vi "laser_controller.vi"() -> ()   [LabVIEW 2014]
uses:
  <vilib>/Instr/_visa.llb/VISA Configure Serial Port (Instr).vi
  <vilib>/FieldPoint/Polymorphic Read.llb/FP Read (Float Array).vi
  <vilib>/FieldPoint/Polymorphic Write.llb/FP Write (Float).vi
panel:
  in  "Ignore Ethernal":bool
  in  "Change Power?":bool
  out "TEC Setpoint":dbl=39.06 format="%#_13g"
  out "Power":dbl(graph)=89.68
  in  "DISABLE":bool
  in  "ENABLE":bool
  in  "LEVEL CONTROL, 0-100 (%)":dbl(knob) scale=0.0..100.0
  out "Temp":dbl(graph)=38.91
  in  "Which Temp?":enum16{"ETH", "PUMP", "PCB", "AMP", "CASE"}(ring)
  out "Temp Stable":bool=TRUE
  out "Software Enabled":bool=TRUE
  out "Hardware Enabled":bool=TRUE
  in  "Ethernal COM Port":refnum<visa-resource-name>="COM3"
  in  "LEVEL CONTROL, 0-10 (W)":dbl(knob) scale=0.0..10.0
  in  "AMPLIFIER ENABLE":bool=TRUE
  out "Pre-amp Mon (Amps)":dbl=5.782406330108643 format="%#_3g"
  out "Temp Mon (deg C)":dbl(slide)=24.883191287517548 scale=0.0..50.0
  out "Mid Power Mon (Volts, no-cal)":dbl=4.550704002380371 format="%#_3g"
  out "Out Power Mon (Volts, no-cal)":dbl=1.5106858015060425 format="%#_3g"
  out "+5 Vdc Out":dbl=4.966402530670166 format="%#_3g"
  out "Power-Amp Pump Current (Amps)":dbl format="%#_3g"
  out "Seed Mon (Volts, no-cal)":dbl=4.966084957122803 format="%#_3g"
  out "Back Refl. Mon (Volts, no-cal)":dbl=0.007061874959617853 format="%#_3g"
  out "Power Supply Fault":bool=TRUE
  out "Temp. Fault":bool=TRUE
  out "Back Refl. Fault":bool=TRUE
  out "Seed Power Fault":bool=TRUE
  out "Master Fault":bool=TRUE
  in  "Controller Stop":bool
  in  "Control Rate (ms)":u32=1000
  # "ORBITS SEED LASER"
  # "NUFERN FIBER AMPLIFIER"
  # "STATUS"
  # "FAULT STATUS"
  # "MONITORS"
  # "OFF STATUS"
  # "ON STATUS"
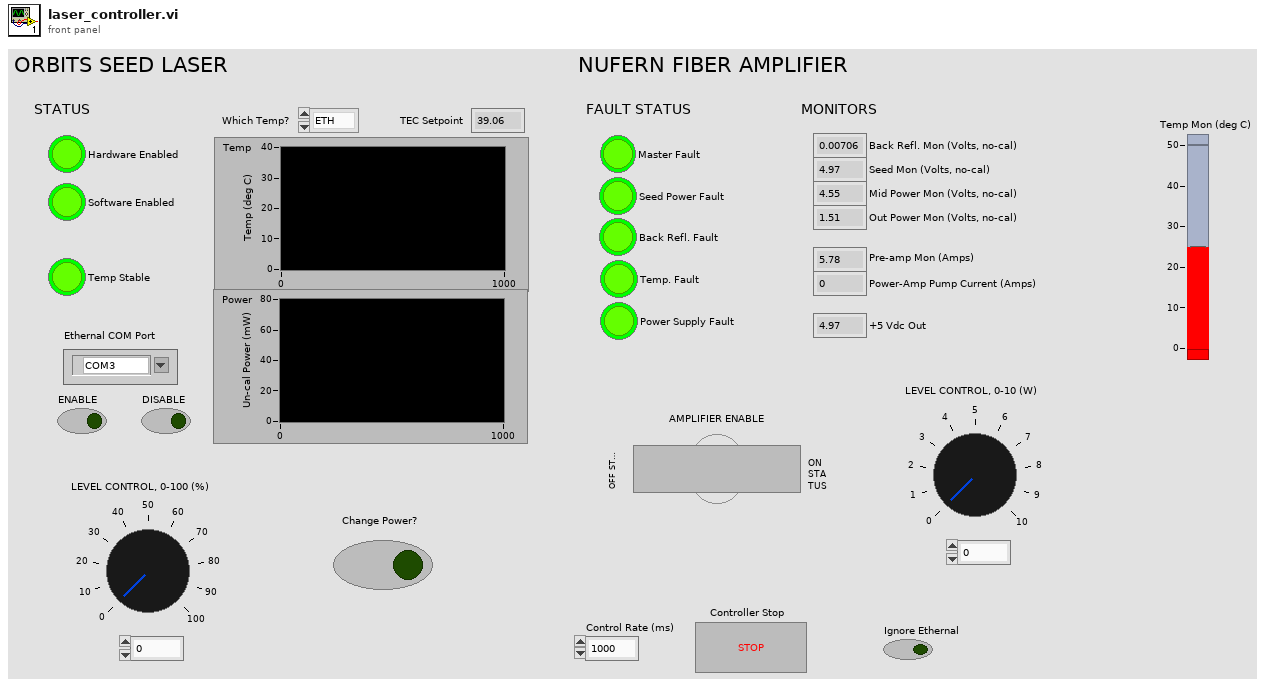
[diagram p1: front panel]
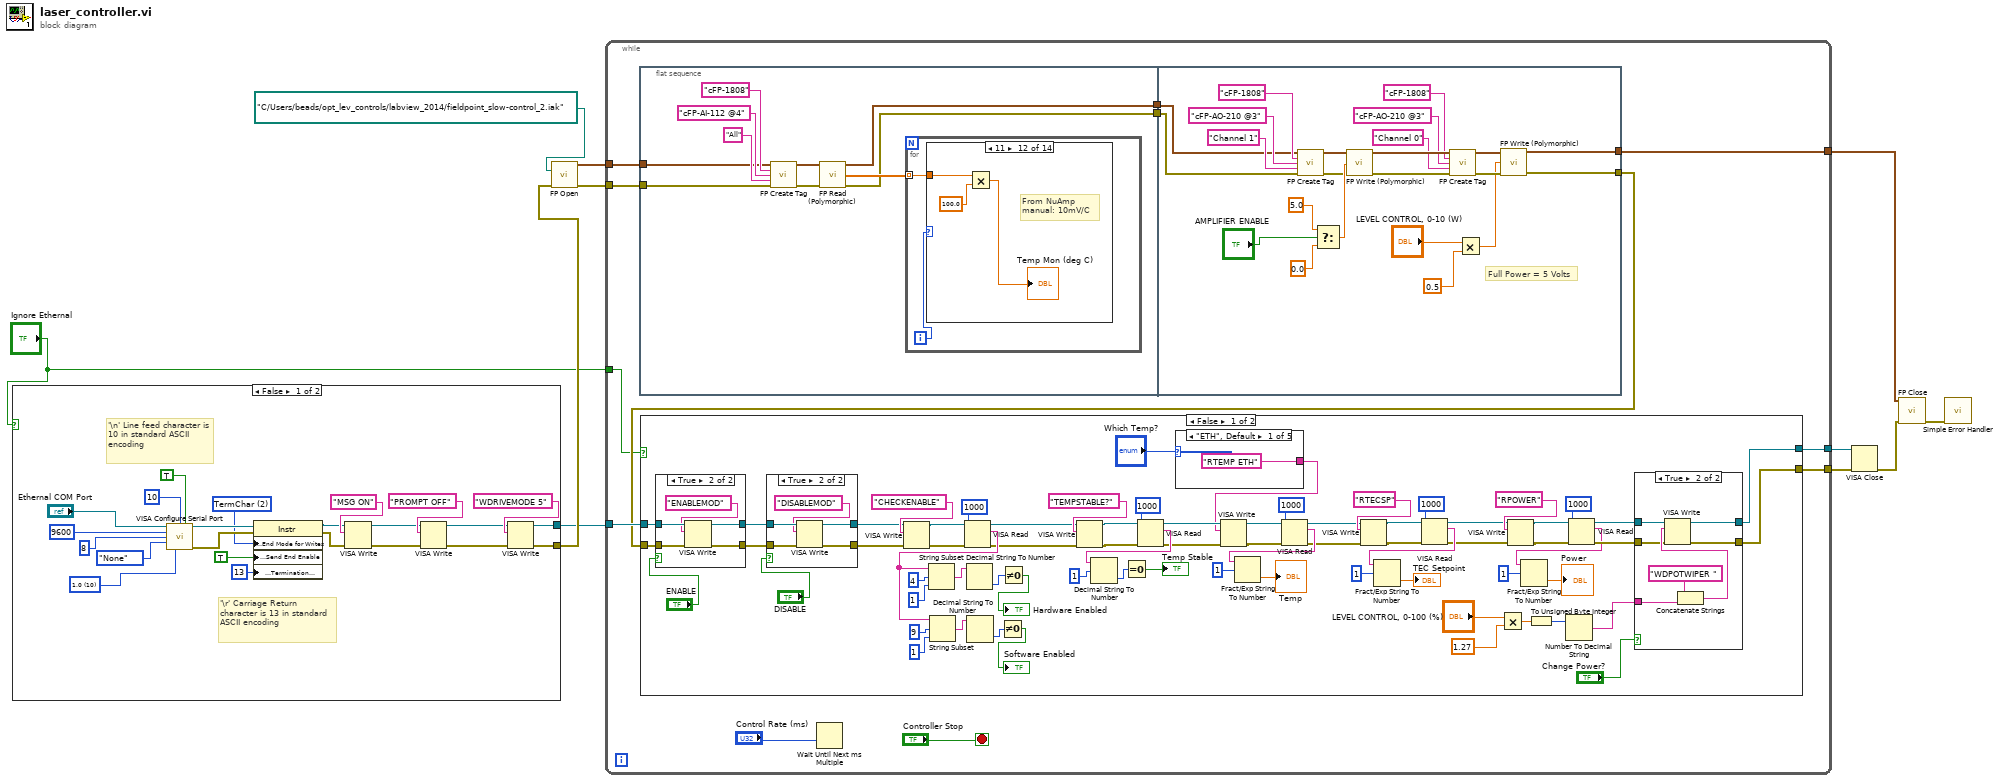
[diagram p0: block diagram]
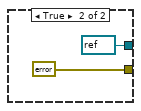
[diagram p2: hidden frame]
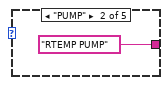
[diagram p6: hidden frame]
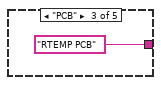
[diagram p7: hidden frame]
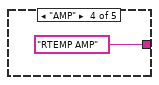
[diagram p8: hidden frame]
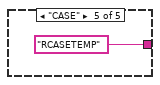
[diagram p9: hidden frame]
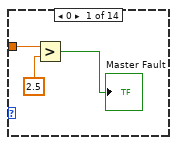
[diagram p11: hidden frame]
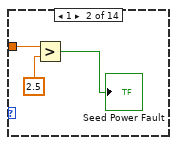
[diagram p12: hidden frame]
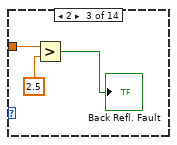
[diagram p13: hidden frame]
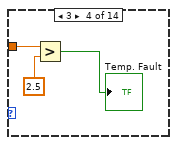
[diagram p14: hidden frame]
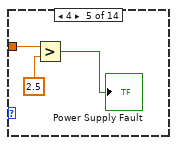
[diagram p15: hidden frame]
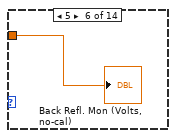
[diagram p16: hidden frame]
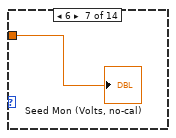
[diagram p17: hidden frame]
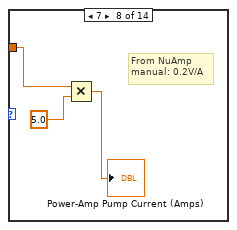
[diagram p18: hidden frame]
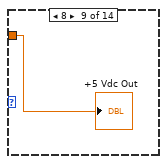
[diagram p19: hidden frame]
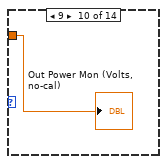
[diagram p20: hidden frame]
diagram:
  n1 = case shown="False" "Ignore Ethernal" {
    tunnel: [w13 errorcluster {"status"=FALSE, "code"=0, "source"=""} ("error out")] -> w3
    tunnel: [w12 refnum<visa-resource-name> refnum ("VISA resource name out")] -> w2
    frame False {
      w17 = u16 10 items=["1.0"=10, "1.5"=15, "2.0"=20] ("stop bits (10: 1 bit)")
      w31 = u16 2 items=["None", "LastBit", "TermChar", "Break"] ("Serial Settings:Serial End Mode for Writes")
      # "'\\r' Carriage Return character is 13 in standard ASCII encoding"
      # "'\\n' Line feed character is 10 in standard ASCII encoding"
      n2 = call-poly "VISA Configure Serial Port"("VISA resource name"="Ethernal COM Port", "termination char\n(0xA = '\\n' = LF)"=u8 10, "Enable Termination\nChar (T)"=TRUE, "baud rate (9600)"=u32 9600, "data bits (8)"=u16 8, "parity (0:none)"=enum16{"None", "Odd", "Even", "Mark", "Space"}."None", "stop bits (10: 1 bit)"=w17) -> ("VISA resource name out"=w33:refnum<visa-resource-name>, "error out"=w34:errorcluster)  [unwired: 3 in, 4 out]
      n3 = property class="Instr"(reference=w33, error in=w34, "Serial Settings:End Mode for Writes"=w31, "Message Based Settings:Send End Enable"=TRUE, "Message Based Settings:Termination Character"=13) -> (reference out=w22:refnum<visa-resource-name>, error out=w23:errorcluster)
      n4 = VISA Write(VISA resource name=w22, write buffer="MSG ON" ("Enable 2"), error in (no error)=w23) -> (VISA resource name out=w20:refnum<visa-resource-name>, error out=w19:errorcluster)  [unwired: 1 out]
      n5 = VISA Write(VISA resource name=w20, write buffer="PROMPT OFF" ("Enable 2"), error in (no error)=w19) -> (VISA resource name out=w15:refnum<visa-resource-name>, error out=w14:errorcluster)  [unwired: 1 out]
      n6 = VISA Write(VISA resource name=w15, write buffer="WDRIVEMODE 5" ("Enable 2"), error in (no error)=w14) -> (VISA resource name out=w12:refnum<visa-resource-name>, error out=w13:errorcluster)  [unwired: 1 out]
    }
    frame True {
    }
  }
  n7 = call <vilib>:"FP Open.vi"("iak file path"=path "C:/Users/beads/opt_lev_controls/labview_2014/fieldpoint_slow-control_2.iak", "error in (no error)"=w3) -> ("FP refnum out"=w11:cluster{"server refnum":u32, "tag refnum":u32}, "error out"=w10:errorcluster)  [unwired: 12 in]
  n8 = while {
    tunnel: w11 -> [w46]
    tunnel: w10 -> [w45]
    tunnel: [w42] -> w8
    tunnel: w2 -> [w39]
    tunnel: [w41] -> w5
    tunnel: [w40] -> w4
    tunnel: "Ignore Ethernal" -> [w37]
    stop <- "Controller Stop" stop-if-true
    n9 = flat-sequence {
      tunnel: w46 -> [w153]
      tunnel: w45 -> [w152]
      tunnel: [w151] -> w44
      tunnel: [w150] -> w43
      tunnel: w44 -> [w210]
      tunnel: w43 -> [w209]
      tunnel: [w195] -> w42
      tunnel: [w194] -> w38
      frame #0 {
        n10 = call <vilib>:"FP Create Tag.vi"("FP refnum in"=w153, "comm resource name"="cFP-1808" ("Comm Resource Name"), "device name"="cFP-AI-112 @4" ("Device Name"), "item name"="All" ("Item Name"), "error in (no error)"=w152) -> ("FP refnum out"=w155:cluster{"server refnum":u32, "tag refnum":u32}, "error out"=w154:errorcluster)  [unwired: 9 in]
        n11 = call-poly <vilib>:"FP Read (Polymorphic).vi"("FP refnum in"=w155, "error in (no error)"=w154) -> ("FP refnum out"=w151:cluster{"server refnum":u32, "tag refnum":u32}, "values"=w159:dbl[], "error out"=w150:errorcluster)  [unwired: 10 in, 1 out]
        n12 = for {
          tunnel: w159 -> [w161] mode=indexing
          i -> [w160]
          n13 = case shown="11" w160 {
            tunnel: w161 -> [w164 w167 w170 w173 w176 w177 w178 w181 w182 w183 w184 w186 w189 _]
            frame 0 {
              n14 = Greater?(x=w164, y=2.5) -> (0:→"Master Fault":bool)
            }
            frame 1 {
              n15 = Greater?(x=w167, y=2.5) -> (0:→"Seed Power Fault":bool)
            }
            frame 2 {
              n16 = Greater?(x=w170, y=2.5) -> (0:→"Back Refl. Fault":bool)
            }
            frame 3 {
              n17 = Greater?(x=w173, y=2.5) -> (0:→"Temp. Fault":bool)
            }
            frame 4 {
              n18 = Greater?(x=w176, y=2.5) -> (0:→"Power Supply Fault":bool)
            }
            frame 5 {
              "Back Refl. Mon (Volts, no-cal)" <- w177
            }
            frame 6 {
              "Seed Mon (Volts, no-cal)" <- w178
            }
            frame 7 {
              # "From NuAmp \nmanual: 0.2V/A"
              n19 = Multiply(x=w181, y=5.0) -> (x*y=→"Power-Amp Pump Current (Amps)":dbl)
            }
            frame 8 {
              "+5 Vdc Out" <- w182
            }
            frame 9 {
              "Out Power Mon (Volts, no-cal)" <- w183
            }
            frame 10 {
              "Mid Power Mon (Volts, no-cal)" <- w184
            }
            frame 11 {
              # "From NuAmp \nmanual: 10mV/C"
              n20 = Multiply(x=w186, y=100.0) -> (x*y=→"Temp Mon (deg C)":dbl)
            }
            frame 12 {
              # "From NuAmp \nmanual: 0.2V/A"
              n21 = Multiply(x=w189, y=5.0) -> (x*y=→"Pre-amp Mon (Amps)":dbl)
            }
            frame 13, Default {
            }
          }
        }
      }
      frame #1 {
        # "Full Power = 5 Volts"
        n22 = call <vilib>:"FP Create Tag.vi"("FP refnum in"=w210, "comm resource name"="cFP-1808" ("Comm Resource Name"), "device name"="cFP-AO-210 @3" ("Device Name"), "item name"="Channel 1" ("Item Name"), "error in (no error)"=w209) -> ("FP refnum out"=w204:cluster{"server refnum":u32, "tag refnum":u32}, "error out"=w203:errorcluster)  [unwired: 9 in]
        n23 = Select(t=5.0, s="AMPLIFIER ENABLE", f=0.0) -> (s? t:f=w205:dbl)
        n24 = call-poly <vilib>:"FP Write (Polymorphic).vi"("FP refnum in"=w204, "value"=w205, "error in (no error)"=w203) -> ("FP refnum out"=w202:cluster{"server refnum":u32, "tag refnum":u32}, "error out"=w201:errorcluster)  [unwired: 10 in, 1 out]
        n25 = call <vilib>:"FP Create Tag.vi"("FP refnum in"=w202, "comm resource name"="cFP-1808" ("Comm Resource Name"), "device name"="cFP-AO-210 @3" ("Device Name"), "item name"="Channel 0" ("Item Name"), "error in (no error)"=w201) -> ("FP refnum out"=w197:cluster{"server refnum":u32, "tag refnum":u32}, "error out"=w196:errorcluster)  [unwired: 9 in]
        n26 = Multiply(x="LEVEL CONTROL, 0-10 (W)", y=0.5) -> (x*y=w191:dbl)
        n27 = call-poly <vilib>:"FP Write (Polymorphic).vi"("FP refnum in"=w197, "value"=w191, "error in (no error)"=w196) -> ("FP refnum out"=w195:cluster{"server refnum":u32, "tag refnum":u32}, "error out"=w194:errorcluster)  [unwired: 10 in, 1 out]
      }
    }
    n28 = case shown="False" w37 {
      tunnel: [w80 w149] -> w41
      tunnel: [w79 w148] -> w40
      tunnel: w39 -> [w78 w149]
      tunnel: w38 -> [w77 w148]
      frame False {
        n29 = case shown="True" "ENABLE" {
          tunnel: w78 -> [w128 w133]
          tunnel: w77 -> [w127 w132]
          tunnel: [w128 w131] -> w76
          tunnel: [w127 w130] -> w75
          frame False {
          }
          frame True {
            n30 = VISA Write(VISA resource name=w133, write buffer="ENABLEMOD" ("Enable 2"), error in (no error)=w132) -> (VISA resource name out=w131:refnum<visa-resource-name>, error out=w130:errorcluster)  [unwired: 1 out]
          }
        }
        n31 = case shown="True" "DISABLE" {
          tunnel: w76 -> [w121 w126]
          tunnel: w75 -> [w120 w125]
          tunnel: [w121 w124] -> w74
          tunnel: [w120 w123] -> w73
          frame False {
          }
          frame True {
            n32 = VISA Write(VISA resource name=w126, write buffer="DISABLEMOD" ("Enable 2"), error in (no error)=w125) -> (VISA resource name out=w124:refnum<visa-resource-name>, error out=w123:errorcluster)  [unwired: 1 out]
          }
        }
        n33 = VISA Write(VISA resource name=w74, write buffer="CHECKENABLE" ("Enable 2"), error in (no error)=w73) -> (VISA resource name out=w117:refnum<visa-resource-name>, error out=w116:errorcluster)  [unwired: 1 out]
        n34 = VISA Read(VISA resource name=w117, byte count=u32 1000 ("Read Count"), error in (no error)=w116) -> (VISA resource name out=w99:refnum<visa-resource-name>, read buffer=w111:string, error out=w98:errorcluster)  [unwired: 1 out]
        n35 = String Subset(string=w111, offset (0)=4, length (rest)=1) -> (substring=w110:string)
        n36 = String Subset(string=w111, offset (0)=9, length (rest)=1) -> (substring=w109:string)
        n37 = Decimal String To Number(string=w110) -> (number=w108:i32)  [unwired: 2 in, 1 out]
        n38 = Decimal String To Number(string=w109) -> (number=w105:i32)  [unwired: 2 in, 1 out]
        n39 = Not Equal To 0?(x=w105) -> (x != 0?=→"Software Enabled":bool)
        n40 = Not Equal To 0?(x=w108) -> (x != 0?=→"Hardware Enabled":bool)
        n41 = VISA Write(VISA resource name=w99, write buffer="TEMPSTABLE?" ("Enable 2"), error in (no error)=w98) -> (VISA resource name out=w102:refnum<visa-resource-name>, error out=w101:errorcluster)  [unwired: 1 out]
        n42 = VISA Read(VISA resource name=w102, byte count=u32 1000 ("Read Count 3"), error in (no error)=w101) -> (VISA resource name out=w91:refnum<visa-resource-name>, read buffer=w100:string, error out=w90:errorcluster)  [unwired: 1 out]
        n43 = Decimal String To Number(string=w100, offset=1) -> (number=w96:i32)  [unwired: 1 in, 1 out]
        n44 = Equal To 0?(x=w96) -> (x = 0?=→"Temp Stable":bool)
        n45 = case shown="\"ETH\", Default" "Which Temp?" {
          tunnel: ["RTEMP ETH" ("Enable 2") "RTEMP PUMP" ("Enable 2") "RTEMP PCB" ("Enable 2") "RTEMP AMP" ("Enable 2") "RCASETEMP" ("Enable 2")] -> w89
          frame "ETH", Default {
          }
          frame "PUMP" {
          }
          frame "PCB" {
          }
          frame "AMP" {
          }
          frame "CASE" {
          }
        }
        n46 = VISA Write(VISA resource name=w91, write buffer=w89, error in (no error)=w90) -> (VISA resource name out=w93:refnum<visa-resource-name>, error out=w92:errorcluster)  [unwired: 1 out]
        n47 = VISA Read(VISA resource name=w93, byte count=u32 1000 ("Read Count 3"), error in (no error)=w92) -> (VISA resource name out=w59:refnum<visa-resource-name>, read buffer=w88:string, error out=w58:errorcluster)  [unwired: 1 out]
        n48 = Fract/Exp String To Number(string=w88, offset=1) -> (number=→"Temp":dbl)  [unwired: 2 in, 1 out]
        n49 = VISA Write(VISA resource name=w59, write buffer="RTECSP" ("Enable 2"), error in (no error)=w58) -> (VISA resource name out=w64:refnum<visa-resource-name>, error out=w63:errorcluster)  [unwired: 1 out]
        n50 = VISA Read(VISA resource name=w64, byte count=u32 1000 ("Read Count 3"), error in (no error)=w63) -> (VISA resource name out=w57:refnum<visa-resource-name>, read buffer=w60:string, error out=w56:errorcluster)  [unwired: 1 out]
        n51 = Fract/Exp String To Number(string=w60, offset=1) -> (number=→"TEC Setpoint":dbl)  [unwired: 2 in, 1 out]
        n52 = Multiply(x="LEVEL CONTROL, 0-100 (%)", y=1.27) -> (x*y=w51:dbl)
        n53 = VISA Write(VISA resource name=w57, write buffer="RPOWER" ("Enable 2"), error in (no error)=w56) -> (VISA resource name out=w85:refnum<visa-resource-name>, error out=w84:errorcluster)  [unwired: 1 out]
        n54 = To Unsigned Byte Integer(number=w51) -> (unsigned 8bit integer=w50:u8)
        n55 = Number To Decimal String(number=w50) -> (decimal integer string=w49:string)  [unwired: 1 in]
        n56 = VISA Read(VISA resource name=w85, byte count=u32 1000 ("Read Count 3"), error in (no error)=w84) -> (VISA resource name out=w82:refnum<visa-resource-name>, read buffer=w67:string, error out=w81:errorcluster)  [unwired: 1 out]
        n57 = Fract/Exp String To Number(string=w67, offset=1) -> (number=→"Power":dbl)  [unwired: 2 in, 1 out]
        n58 = case shown="True" "Change Power?" {
          tunnel: w49 -> [_ w141]
          tunnel: w82 -> [w135 w139]
          tunnel: w81 -> [w134 w138]
          tunnel: [w135 w137] -> w80
          tunnel: [w134 w136] -> w79
          frame False {
          }
          frame True {
            n59 = Concatenate Strings("WDPOTWIPER " ("Enable 2"), w141) -> (w140:string)
            n60 = VISA Write(VISA resource name=w139, write buffer=w140, error in (no error)=w138) -> (VISA resource name out=w137:refnum<visa-resource-name>, error out=w136:errorcluster)  [unwired: 1 out]
          }
        }
      }
      frame True {
      }
    }
    n61 = Wait Until Next ms Multiple(millisecond multiple="Control Rate (ms)") -> ()  [unwired: 1 out]
  }
  n62 = VISA Close(VISA resource name=w5, error in (no error)=w4) -> (error out=w6:errorcluster)
  n63 = call <vilib>:"FP Close.vi"("FP refnum in"=w8, "error in (no error)"=w6) -> ("error out"=w9:errorcluster)  [unwired: 13 in]
  n64 = call <vilib>:"Simple Error Handler.vi"("error in (no error)"=w9) -> ()  [unwired: 4 in, 5 out]
